vi "Tiempo continuo Versión 3.vi"() -> ()   [LabVIEW 2018]
uses:
  <vilib>/addons/control/pid/NI_PID_pid.lvlib
  <vilib>/addons/control/pid/pid.llb/PID (DBL).vi
  <vilib>/Analysis/Matrix/Datatypes/RealMatrix.ctl
  <vilib>/Analysis/Matrix/NI_Matrix.lvlib
panel:
  in  "PID gains":T1={"proportional gain (Kc)"=1.0, "integral time (Ti, min)"=0.01, "derivative time (Td, min)"=0.0} {"derivative time (Td, min)" format="%.3f"; "integral time (Ti, min)" format="%.3f"; "proportional gain (Kc)" format="%.3f"}
  in  "Retardo":dbl format="%.2f segundos"
  in  "Denominador":dbl[](array[numeric])
  in  "Numerador":dbl[](array[numeric])
  out "Ley de Control":dbl
  in  "Lazo":bool
  out "Grafica":T2(graph)
  in  "stop":bool
  out "y(t)":dbl
  in  "setpoint":dbl(slide) scale=0.0..100.0
  out "B":dbl[](array[numeric])=[1.0, 0.0]
  out "C":dbl[](array[numeric])=[1.0, 2.0]
  out "A":T3=[[-2.0, -1.0], [1.0, 0.0]]
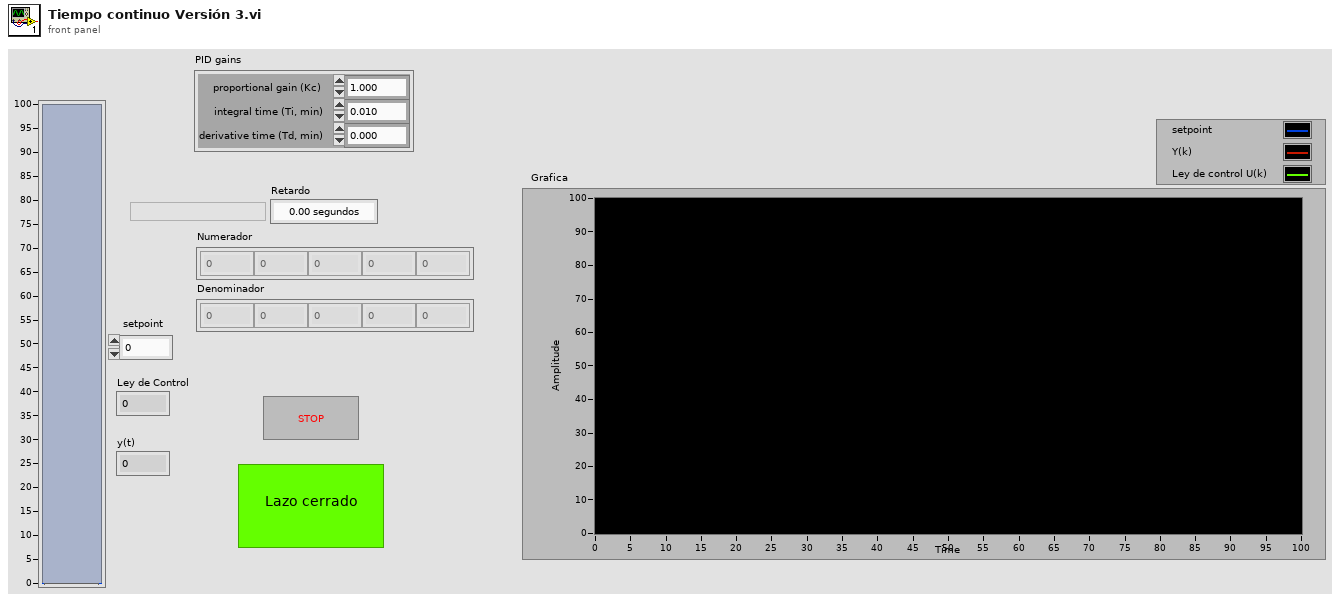
[diagram p1: front panel]
types:
  T1 = cluster{"proportional gain (Kc)":dbl, "integral time (Ti, min)":dbl, "derivative time (Td, min)":dbl}
  T2 = cluster{"setpoint":dbl, "y(k)":dbl, "Ley de Control":dbl}
  T3 = typedef "NI_Matrix.lvlib/RealMatrix.ctl" = dbl[][]
  T4 = cluster{"setpoint":dbl, "y(k)":dbl, "Ley de Control":dbl}[]
  T5 = cluster{"setpoint":dbl, "y(t)":dbl, "Ley de Control":dbl}
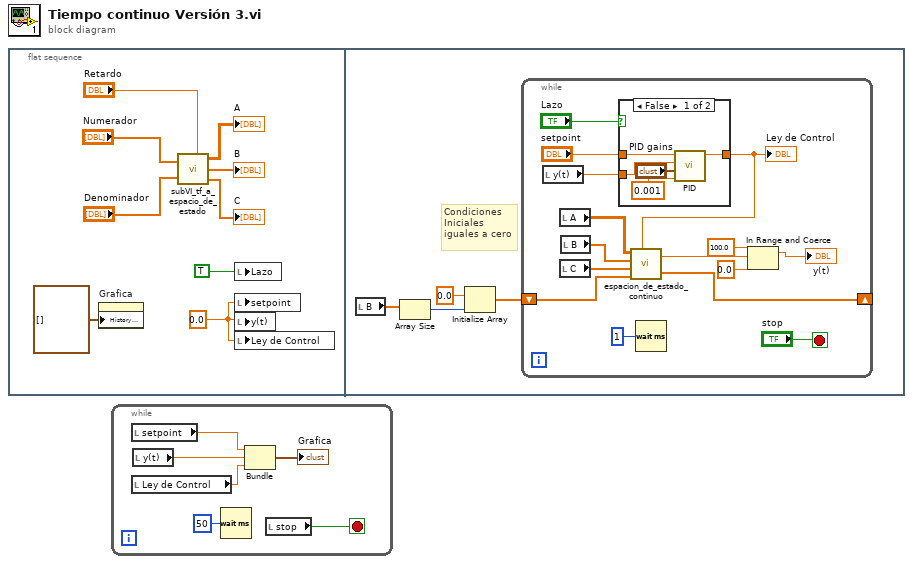
[diagram p0: block diagram]
diagram:
  n1 = flat-sequence {
    frame #0 {
      w2 = 0.0
      n2 = property on="Grafica" class="WFChart (strict)"("History Data"=T4 []) -> ()  [unwired: 2 in, 2 out]
      n3 = call "subVI_tf_a_espacio_de_estado.vi"("Retardo"="Retardo", "Denominador"="Denominador", "Numerador"="Numerador") -> ("C"=→"C":dbl[], "B"=→"B":dbl[], "A"=→"A":T3)  [unwired: 1 in]
      n4 = local write "Lazo"(TRUE ("Lazo")) -> ()
      n5 = local write "setpoint"(w2) -> ()
      n6 = local write "y(t)"(w2) -> ()
      n7 = local write "Ley de Control"(w2) -> ()
    }
    frame #1 {
      # "Condiciones\nIniciales\niguales a cero"
      n8 = local read "B"() -> (w13:dbl[])
      n9 = Array Size(array=w13) -> (size(s)=w11:i32)
      n10 = Initialize Array(0.0 ("element"), w11) -> (w12:dbl[])
      n11 = while {
        shift-right: [w22] -> _
        shift-left: w12 -> [w18]
        stop <- "stop" stop-if-true
        n12 = local read "y(t)"() -> (w21:dbl)
        n13 = local read "A"() -> (w25:T3)
        n14 = local read "C"() -> (w23:dbl[])
        n15 = local read "B"() -> (w24:dbl[])
        n16 = case shown="False" "Lazo" {
          tunnel: [w32 w34] -> w20
          tunnel: "setpoint" -> [w33 w34]
          tunnel: w21 -> [w31 _]
          frame False {
            n17 = call-poly <vilib>:"PID.vi"("dt (s)"=0.001, "PID gains"="PID gains", "process variable"=w31, "setpoint"=w33) -> ("output"=w32:dbl)  [unwired: 6 in, 1 out]
          }
          frame True {
            # "toma como\nreferencia sp"
            # "Lazo\nabierto"
          }
        }
        "Ley de Control" <- w20
        n18 = call "espacion_de_estado_continuo.vi"("A"=w25, "B"=w24, "C"=w23, "dX(t)"=w18, "u(t)"=w20) -> ("y(t)"=w15:dbl, "X(t)"=w22:dbl[])
        n19 = Wait (ms)(milliseconds to wait=1) -> ()  [unwired: 1 out]
        n20 = In Range and Coerce(upper limit=100.0, x=w15, lower limit=0.0) -> (coerced(x)=→"y(t)":dbl)  [unwired: 1 out]
      }
    }
  }
  n21 = while {
    stop <- w40 stop-if-true
    n22 = local read "setpoint"() -> (w37:dbl)
    n23 = local read "Ley de Control"() -> (w35:dbl)
    n24 = local read "y(t)"() -> (w36:dbl)
    n25 = Wait (ms)(milliseconds to wait=u32 50) -> ()  [unwired: 1 out]
    n26 = Bundle("setpoint"=w37, "y(t)"=w36, "Ley de Control"=w35) -> (→"Grafica":T5)  [unwired: 1 in]
    n27 = local read "stop"() -> (w40:bool)
  }
